vi "LV cRIO.vi"() -> ()   [LabVIEW 2025]
uses:
  <vilib>/measure/NI_MABase.lvlib
panel:
  out "Signal":waveform(dbl)(graph)={"t0"=timestamp(0 s since 1904-01-01), "dt"=0.0001, "Y"=[]}
  in  "Amplitude":dbl=0.5
  in  "Frequency":dbl=400.0
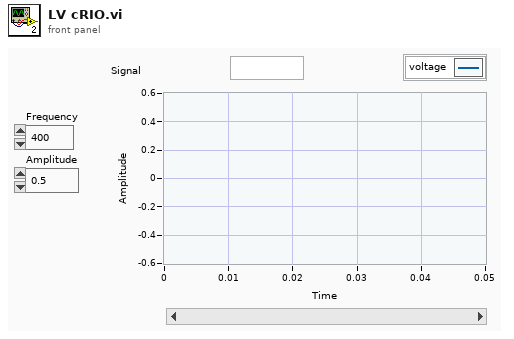
[diagram p1: front panel]
types:
  T1 = enum16{"Sine Wave", "Triangle Wave", "Square Wave", "Sawtooth Wave"}
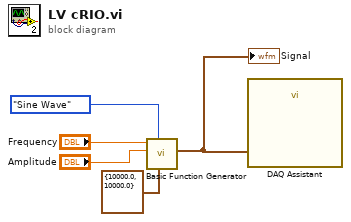
[diagram p0: block diagram]
diagram:
  n1 = call <vilib>:"Basic Function Generator.vi"("sampling info"=cluster{"Fs":dbl, "#s":dbl} {"Fs"=10000.0, "#s"=10000.0}, "signal type"=T1."Sine Wave", "amplitude"="Amplitude", "frequency"="Frequency") -> ("signal out"=w2:waveform(dbl))  [unwired: 5 in, 2 out]
  "Signal" <- w2
  n2 = call "DAQ Assistant"("data"=w2) -> ()  [unwired: 17 in, 2 out]
